vi "TrendsD27.vi"() -> ()   [LabVIEW 2019, in "D02.lvlib"]
uses:
  D02.lvlib
panel:
  out "No Change":bool
  out "Sudden Change":bool
  out "Decrease":bool
  out "Increase":bool
  out "Previous  ES":dbl
  out "Present  Speed":dbl
  out "Present Error":dbl format="%#.2g"
  out "Previous Error":dbl
  out "Previous  Speed":dbl
  out "Previous PW":dbl caption="Control Information"
  out "Pulse Trends":waveform(i16)[](graph) caption="Waveform Chart - Dark"
  in  "Close":bool
  out "disc name":string="Disc 27 Trends"
  out "dsgs":string="DSGS"
  out "Speed Trend":waveform(dbl)(graph) caption="Waveform Chart - Dark"
  out "Average Trend":waveform(dbl)[](graph) caption="Waveform Chart - Dark"
  out "Live Trend":waveform(dbl)[](graph) caption="Waveform Chart - Dark"
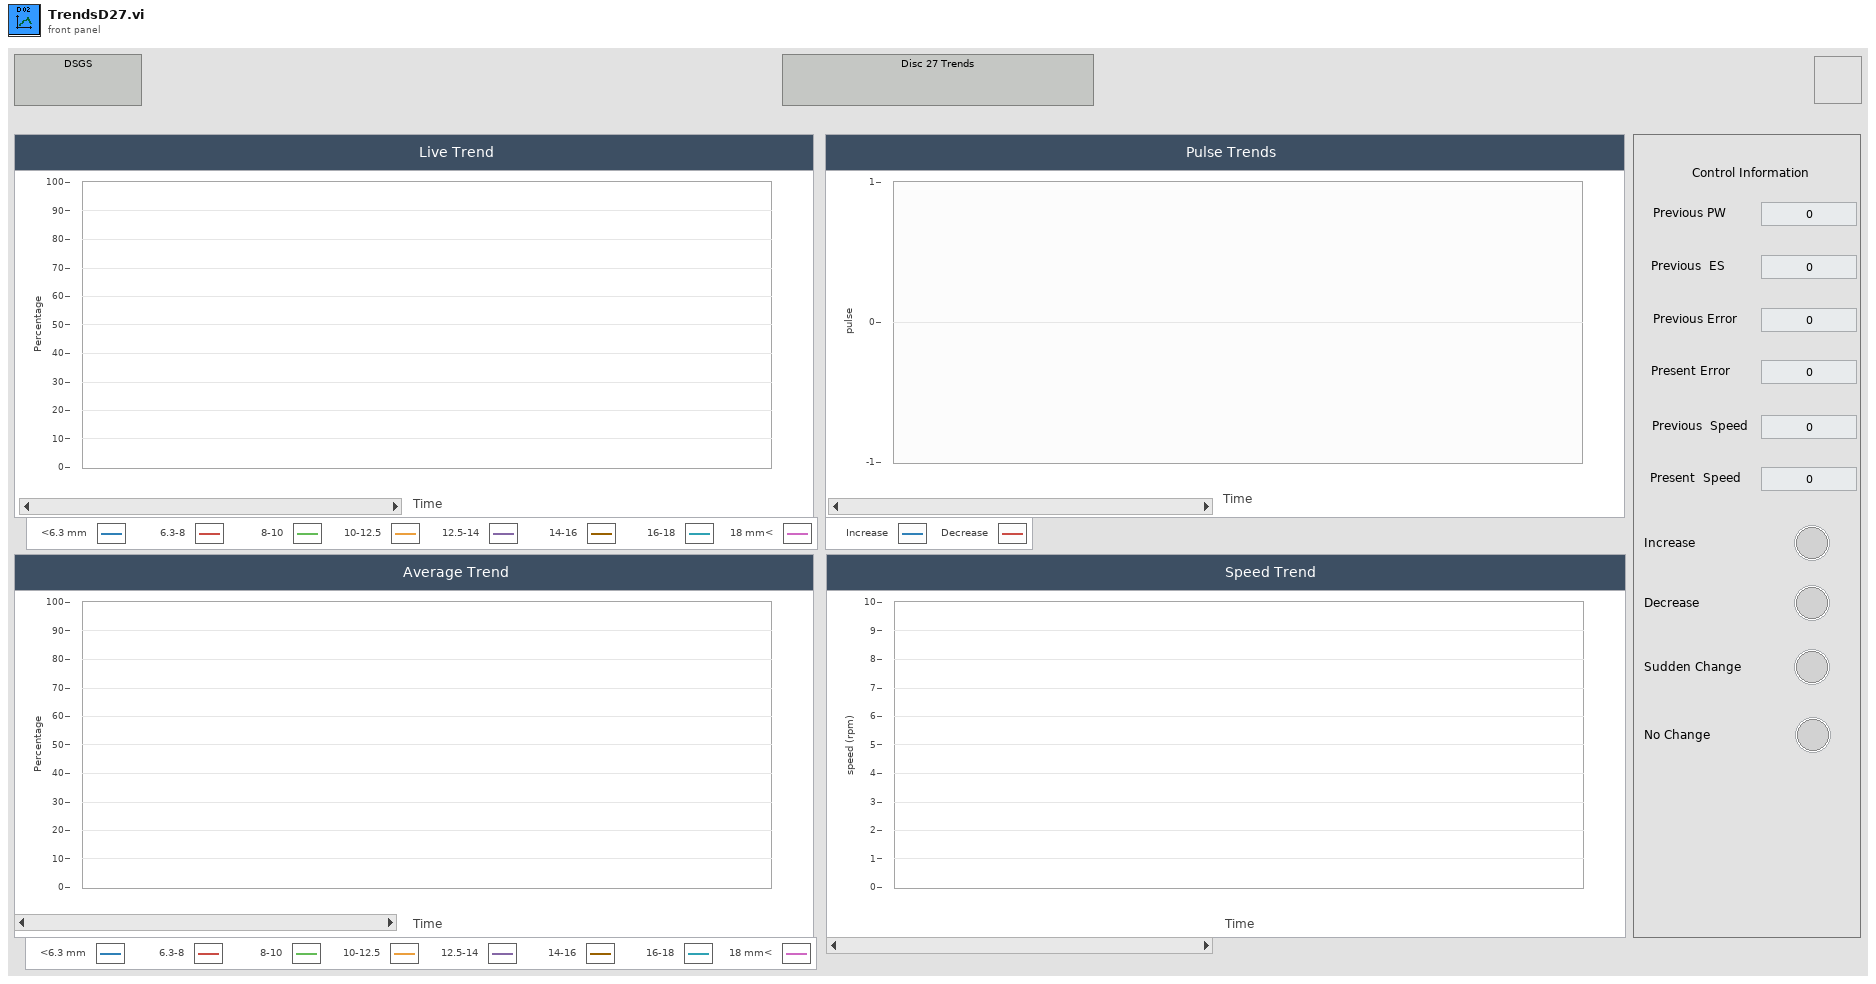
[diagram p1: front panel]
types:
  T1 = cluster{"decrease D27":bool, "increase D27":bool, "no change D27":bool, "sudden change D27":bool, "last error 27":dbl, "previous speed D27":dbl, "pulse width D27":dbl, "slope D27":dbl}
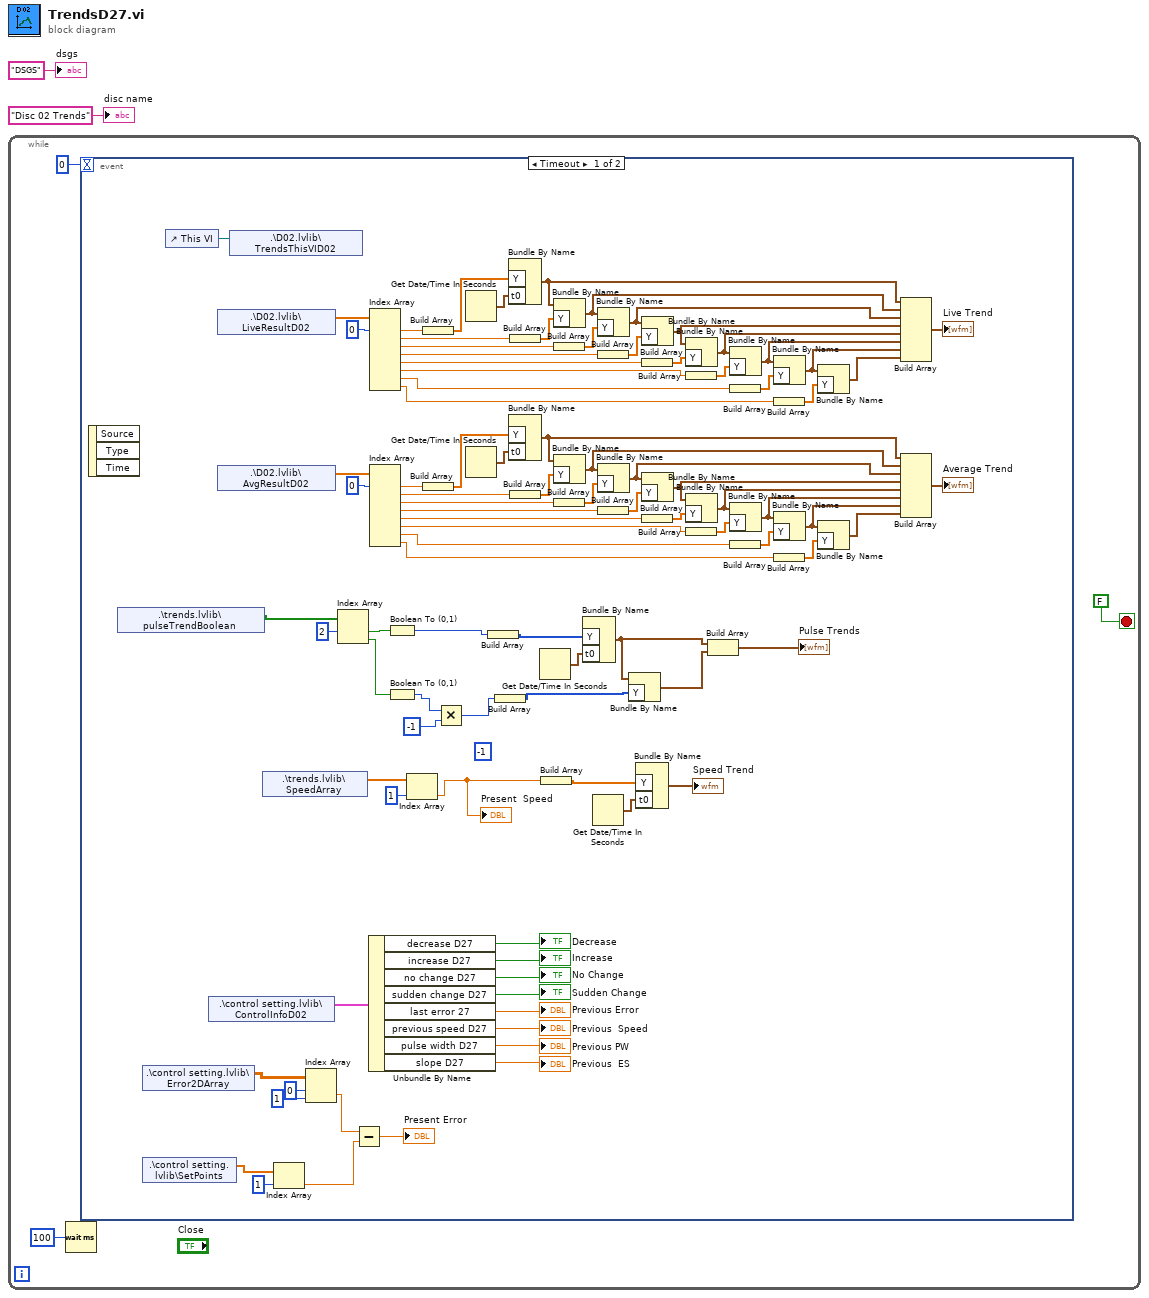
[diagram p0: block diagram]
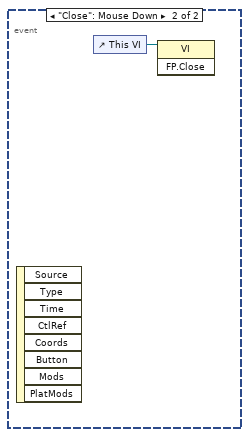
[diagram p2: hidden frame]
diagram:
  n1 = while {
    stop <- FALSE stop-if-true
    n2 = Wait (ms)(milliseconds to wait=u32 100) -> ()  [unwired: 1 out]
    n3 = event shown="[0] Timeout" {
      selector: _ -> [_ _]
      dyn-events: _ -> [_ _]
      timeout: 0 -> [_ _]
      event Timeout {
        (unwired) i16 -1 ("0, 1")
        n4 = event-data() -> ()  [unwired: 1 in, 3 out]
        n5 = shared-variable ".\\trends.lvlib\\pulseTrendBoolean"() -> (w39:bool[])  [unwired: 1 in, 1 out]
        n6 = shared-variable ".\\control setting.lvlib\\Error2DArray"() -> (w14:dbl[][])  [unwired: 1 in, 1 out]
        n7 = shared-variable ".\\control setting.lvlib\\SetPoints"() -> (w11:dbl[])  [unwired: 1 in, 1 out]
        n8 = control-ref of="This VI"() -> (w43:refnum<vi>)
        n9 = shared-variable ".\\control setting.lvlib\\ControlInfoD02"() -> (w23:T1)  [unwired: 1 in, 1 out]
        n10 = shared-variable ".\\D02.lvlib\\LiveResultD02"() -> (w99:dbl[])  [unwired: 1 in, 1 out]
        n11 = shared-variable ".\\D02.lvlib\\AvgResultD02"() -> (w54:dbl[])  [unwired: 1 in, 1 out]
        n12 = shared-variable ".\\D02.lvlib\\TrendsThisVID02"(w43) -> ()  [unwired: 1 in, 1 out]
        n13 = shared-variable ".\\trends.lvlib\\SpeedArray"() -> (w28:dbl[])  [unwired: 1 in, 1 out]
        n14 = Index Array(array=w11, index=1) -> (element=w8:dbl)
        n15 = Index Array(array=w14, index (row)=0, index (col)=1 ("disabled index (col)")) -> (element=w9:dbl)
        n16 = Index Array(array=w39, index #1=2 ("index")) -> (element #1=w38:bool, element #2=w36:bool)  [unwired: 1 in]
        n17 = Subtract(x=w9, y=w8) -> (x-y=→"Present Error":dbl)
        n18 = Unbundle By Name(w23) -> ("decrease D27"=→"Decrease":bool, "increase D27"=→"Increase":bool, "no change D27"=→"No Change":bool, "sudden change D27"=→"Sudden Change":bool, "last error 27"=→"Previous Error":dbl, "previous speed D27"=→"Previous  Speed":dbl, "pulse width D27"=→"Previous PW":dbl, "slope D27"=→"Previous  ES":dbl)
        n19 = Index Array(array=w99, index #1=0 ("index")) -> (element #1=w89:dbl, element #2=w88:dbl, element #3=w86:dbl, element #4=w84:dbl, element #5=w83:dbl, element #6=w81:dbl, element #7=w79:dbl, element #8=w50:dbl)  [unwired: 7 in]
        n20 = Index Array(array=w54, index #1=0 ("index")) -> (element #1=w64:dbl, element #2=w65:dbl, element #3=w67:dbl, element #4=w69:dbl, element #5=w70:dbl, element #6=w72:dbl, element #7=w74:dbl, element #8=w46:dbl)  [unwired: 7 in]
        n21 = Boolean To (0,1)(Boolean=w38) -> (0, 1=w37:i16)
        n22 = Boolean To (0,1)(Boolean=w36) -> (0, 1=w32:i16)
        n23 = Index Array(array=w28, index=1) -> (element=w6:dbl)
        "Present  Speed" <- w6
        n24 = Build Array(w89) -> (w78:dbl[])
        n25 = Build Array(w64) -> (w75:dbl[])
        n26 = Multiply(x=w32, y=i16 -1 ("0, 1")) -> (x*y=w30:i16)
        n27 = Get Date/Time In Seconds() -> (seconds since 1Jan1904=w96:timestamp)
        n28 = Get Date/Time In Seconds() -> (seconds since 1Jan1904=w57:timestamp)
        n29 = Build Array(w37) -> (w40:i16[])
        n30 = Build Array(w30) -> (w35:i16[])
        n31 = Bundle By Name("Y"=w78, "t0"=w96) -> (w90:waveform(dbl))  [unwired: 1 in]
        n32 = Bundle By Name("Y"=w75, "t0"=w57) -> (w63:waveform(dbl))  [unwired: 1 in]
        n33 = Build Array(w88) -> (w87:dbl[])
        n34 = Build Array(w65) -> (w66:dbl[])
        n35 = Get Date/Time In Seconds() -> (seconds since 1Jan1904=w41:timestamp)
        n36 = Build Array(w6) -> (w26:dbl[])
        n37 = Bundle By Name(cluster=w90, "Y"=w87) -> (w91:waveform(dbl))
        n38 = Build Array(w86) -> (w85:dbl[])
        n39 = Bundle By Name(cluster=w63, "Y"=w66) -> (w62:waveform(dbl))
        n40 = Build Array(w67) -> (w68:dbl[])
        n41 = Bundle By Name("Y"=w40, "t0"=w41) -> (w34:waveform(i16))  [unwired: 1 in]
        n42 = Get Date/Time In Seconds() -> (seconds since 1Jan1904=w25:timestamp)
        n43 = Bundle By Name(cluster=w91, "Y"=w85) -> (w92:waveform(dbl))
        n44 = Build Array(w84) -> (w97:dbl[])
        n45 = Bundle By Name(cluster=w62, "Y"=w68) -> (w61:waveform(dbl))
        n46 = Build Array(w69) -> (w56:dbl[])
        n47 = Bundle By Name(cluster=w34, "Y"=w35) -> (w33:waveform(i16))
        n48 = Bundle By Name("Y"=w26, "t0"=w25) -> (→"Speed Trend":waveform(dbl))  [unwired: 1 in]
        n49 = Bundle By Name(cluster=w92, "Y"=w97) -> (w93:waveform(dbl))
        n50 = Build Array(w83) -> (w82:dbl[])
        n51 = Bundle By Name(cluster=w61, "Y"=w56) -> (w60:waveform(dbl))
        n52 = Build Array(w70) -> (w71:dbl[])
        n53 = Bundle By Name(cluster=w93, "Y"=w82) -> (w94:waveform(dbl))
        n54 = Build Array(w81) -> (w80:dbl[])
        n55 = Bundle By Name(cluster=w60, "Y"=w71) -> (w59:waveform(dbl))
        n56 = Build Array(w72) -> (w73:dbl[])
        n57 = Build Array(w34, w33) -> (→"Pulse Trends":waveform(i16)[])
        n58 = Bundle By Name(cluster=w94, "Y"=w80) -> (w95:waveform(dbl))
        n59 = Build Array(w79) -> (w77:dbl[])
        n60 = Bundle By Name(cluster=w59, "Y"=w73) -> (w58:waveform(dbl))
        n61 = Build Array(w74) -> (w76:dbl[])
        n62 = Bundle By Name(cluster=w95, "Y"=w77) -> (w48:waveform(dbl))
        n63 = Build Array(w50) -> (w51:dbl[])
        n64 = Bundle By Name(cluster=w58, "Y"=w76) -> (w44:waveform(dbl))
        n65 = Build Array(w46) -> (w47:dbl[])
        n66 = Bundle By Name(cluster=w48, "Y"=w51) -> (w49:waveform(dbl))
        n67 = Bundle By Name(cluster=w44, "Y"=w47) -> (w45:waveform(dbl))
        n68 = Build Array(w90, w91, w92, w93, w94, w95, w48, w49) -> (→"Live Trend":waveform(dbl)[])
        n69 = Build Array(w63, w62, w61, w60, w59, w58, w44, w45) -> (→"Average Trend":waveform(dbl)[])
      }
      event "Close": Mouse Down {
        n70 = event-data() -> ()  [unwired: 1 in, 8 out]
        n71 = control-ref of="This VI"() -> (w100:refnum<vi>)
        n72 = invoke class="VI" method="FP.Close"(reference=w100) -> ()  [unwired: 2 in, 3 out]
      }
    }
  }
  "dsgs" <- "DSGS" ("dsgs")
  "disc name" <- "Disc 02 Trends" ("disc name")
